vi "Initialize.vi"(8 "error in (no error)":errorcluster, 11 "NIScope in":refnum<class "NIScope.lvclass">) -> (0 "error out":errorcluster, 3 "NIScope out":refnum<class "NIScope.lvclass">)   [LabVIEW 2018, in "ScopePlugins.lvlib" / "NIScope.lvclass"]
doc: "Establishes communication to the scope instrument."
uses:
  NIScope.lvclass
  C:/Users/Public/Projects/ICDAS/NistPluggableModules/Scope/ScopePlugins/ScopePluginBaseClass/ScopePluginsBase.lvclass
  Typedefs/ConnectionArray.ctl
  ScopePluginBaseClass/ScopePluginsBase.lvclass/ScopePluginsBase.ctl
  ScopePluginBaseClass/Accessors/Read Channels.vi
  ScopePluginBaseClass/Accessors/Write Channels.vi
  ScopePluginBaseClass/ScopePluginsBase.lvclass
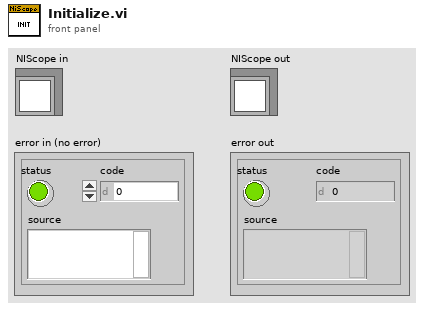
[diagram p1: front panel]
types:
  T1 = typedef "ScopePlugins.lvlib/NIScope.lvclass/ConnectionArray.ctl" = cluster{"Open Connection":bool, "Instrument handle":refnum<k15>}[]
  T2 = typedef "ScopePlugins.lvlib/ScopePluginsBase.lvclass/ChannelSetting(s).ctl" = cluster{"Number of Channels":i32, "Channel(s)":cluster{"Enabled":bool, "Instrument Handle":string, "Channel Name":string, "Maximum Input Frequency":dbl, "Verticle Settings":cluster{"Vertical Range":dbl, "Vertical Offset":dbl, "Probe Attenuation":dbl, "Vertical Coupling":i32}, "Connected":bool, "Input Impedance":dbl, "IO Type Instrument Handle":refnum<k15>}[]}
  T3 = typedef "ScopePlugins.lvlib/ScopePluginsBase.lvclass/InitializationSettings.ctl" = cluster{"Reset":bool, "IdQuery":bool, "AutoConfig":bool, "Options String":string, "Synchronize":bool}
  T4 = cluster{"Enabled":bool, "Instrument Handle":string, "Channel Name":string, "Maximum Input Frequency":dbl, "Verticle Settings":cluster{"Vertical Range":dbl, "Vertical Offset":dbl, "Probe Attenuation":dbl, "Vertical Coupling":i32}, "Connected":bool, "Input Impedance":dbl, "IO Type Instrument Handle":refnum<k15>}[]
  T5 = cluster{"Open Connection":bool, "Instrument handle":refnum<k15>}
  T6 = cluster{"Enabled":bool, "Instrument Handle":string, "Channel Name":string, "Maximum Input Frequency":dbl, "Verticle Settings":cluster{"Vertical Range":dbl, "Vertical Offset":dbl, "Probe Attenuation":dbl, "Vertical Coupling":i32}, "Connected":bool, "Input Impedance":dbl, "IO Type Instrument Handle":refnum<k15>}
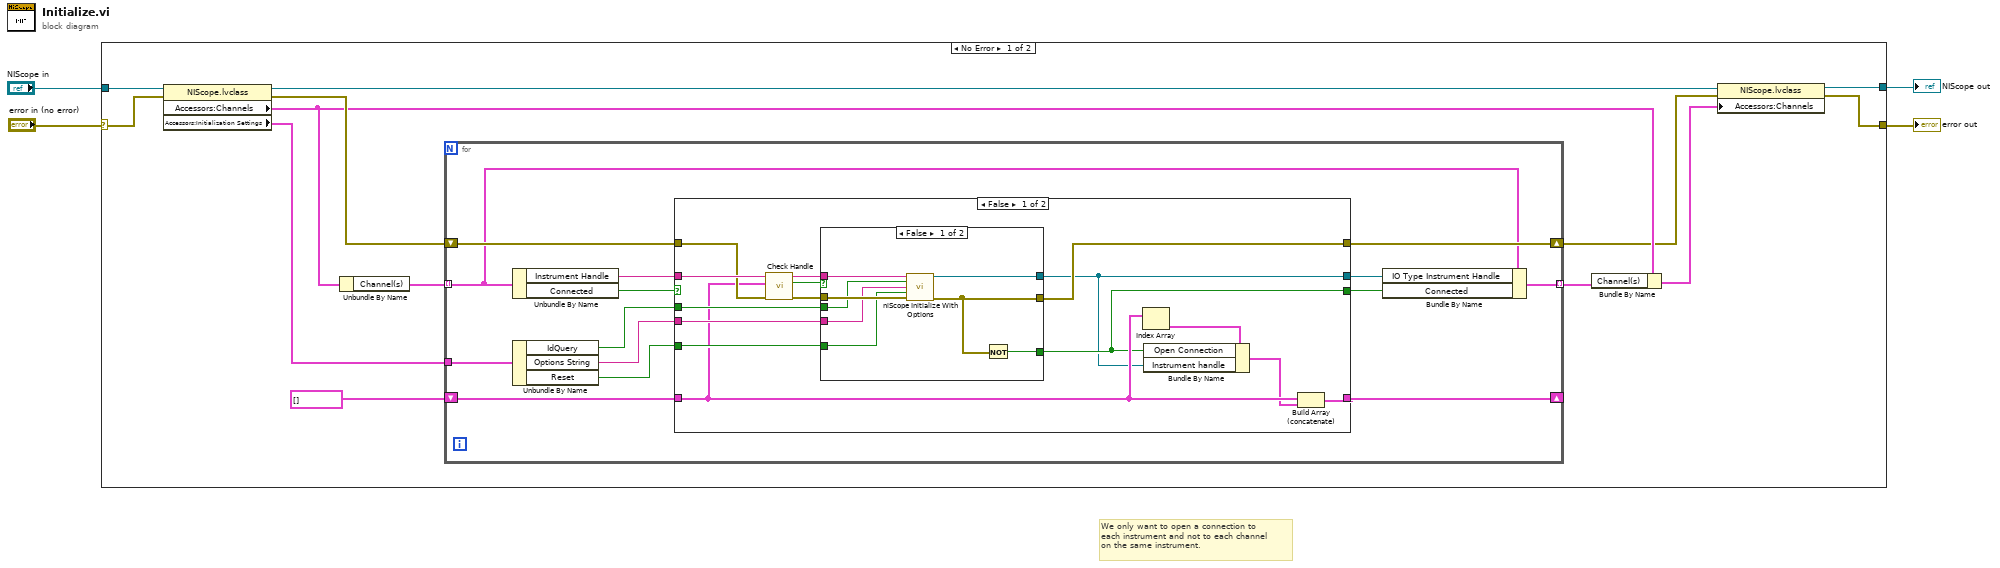
[diagram p0: block diagram]
diagram:
  # "We only want to open a connection to\neach instrument and not to each channel\non the same instrument."
  n1 = case shown="No Error" "error in (no error)" {
    selector: "error in (no error)" -> [w17 w62]
    tunnel: "NIScope in" -> [w7 w63]
    tunnel: [w10 w63] -> w2
    tunnel: [w11 w62] -> w1
    frame No Error {
      n2 = property class="NIScope.lvclass"(reference=w7, error in=w17) -> (reference out=w9:refnum<class "NIScope.lvclass">, error out=w15:errorcluster, "Accessors:Channels"=w13:T2, "Accessors:Initialization Settings"=w5:T3)
      n3 = Unbundle By Name(w13) -> ("Channel(s)"=w16:T4)
      n4 = for {
        tunnel: w16 -> [w26] mode=indexing
        shift-right: [w28] -> w8
        shift-left: w15 -> [w31]
        shift-right: [w29] -> _
        shift-left: T1 [] ("Connection Array") -> [w30]
        tunnel: [w27] -> w14 mode=indexing
        tunnel: w5 -> [w25]
        n5 = Unbundle By Name(w26) -> ("Instrument Handle"=w21:string, "Connected"=w24:bool)
        n6 = Unbundle By Name(w25) -> ("IdQuery"=w18:bool, "Options String"=w19:string, "Reset"=w20:bool)
        n7 = case shown="False" w24 {
          selector: w24 -> [_ w60]
          tunnel: w31 -> [w39 w61]
          tunnel: w21 -> [w41 w59]
          tunnel: w18 -> [w46 _]
          tunnel: w20 -> [w45 _]
          tunnel: w30 -> [w36 w58]
          tunnel: [w34 w60] -> w23
          tunnel: [w32 w59] -> w22
          tunnel: [w44 w58] -> w29
          tunnel: [w43 w61] -> w28
          tunnel: w19 -> [w42 _]
          frame False {
            n8 = call "Check Handle.vi"("error in (no error)"=w39, "Connection Array"=w36, "Handle In"=w41) -> ("error out"=w38:errorcluster, "Duplicate Instrument?"=w37:bool, "Handle Out"=w40:string)  [unwired: 6 in]
            n9 = case shown="False" w37 {
              selector: w37 -> [_ w55]
              tunnel: w38 -> [w54 w57]
              tunnel: [w48 w57] -> w43
              tunnel: [w52 w56] -> w32
              tunnel: w46 -> [w49 _]
              tunnel: w45 -> [w53 _]
              tunnel: [w47 w55] -> w34
              tunnel: w42 -> [w51 _]
              tunnel: w40 -> [w50 w56]
              frame False {
                n10 = call <instrlib>:"niScope Initialize With Options.vi"("resource name"=w50, "id query"=w49, "option string"=w51, "reset device"=w53, "error in"=w54) -> ("instrument handle"=w52:refnum<k15>, "error out"=w48:errorcluster)  [unwired: 9 in]
                n11 = Not(x=w48) -> (.not. x?=w47:bool)
              }
              frame True {
              }
            }
            n12 = Index Array(array=w36) -> (element=w35:T5)  [unwired: 1 in]
            n13 = Bundle By Name(cluster=w35, "Open Connection"=w34, "Instrument handle"=w32) -> (w33:T5)
            n14 = Build Array (concatenate)(w36, w33) -> (w44:T1)
          }
          frame True {
          }
        }
        n15 = Bundle By Name(cluster=w26, "IO Type Instrument Handle"=w22, "Connected"=w23) -> (w27:T6)
      }
      n16 = Bundle By Name(cluster=w13, "Channel(s)"=w14) -> (w12:T2)
      n17 = property class="NIScope.lvclass"(reference=w9, error in=w8, "Accessors:Channels"=w12) -> (reference out=w10:refnum<class "NIScope.lvclass">, error out=w11:errorcluster)
    }
    frame Error {
    }
  }
  "error out" <- w1
  "NIScope out" <- w2
